vi "3.1.13-Ignore Low Values.vi"(1 "Numeric":dbl) -> (0 "t":dbl format="%#_12e")   [LabVIEW 2010]
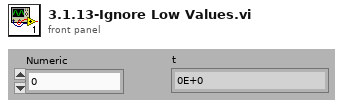
[diagram p1: front panel]
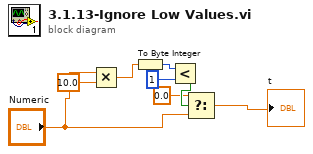
[diagram p0: block diagram]
diagram:
  n1 = Multiply(x="Numeric", y=10.0) -> (x*y=w5:dbl)
  n2 = To Byte Integer(number=w5) -> (8bit integer=w4:i8)
  n3 = Less?(x=w4, y=i8 1) -> (x < y?=w2:bool)
  n4 = Select(t=0.0, s=w2, f="Numeric") -> (s? t:f=→"t":dbl)
